vi "Add CSM Module.vi"(6 "Config Path":path, 8 "error in (no error)":errorcluster, 10 "CSM-VI":string, 11 "CSM Name":string) -> (0 "error out":errorcluster)   [LabVIEW 2017, in "CSM-Helper API with lvcsm Support.lvlib"]
uses:
  CSM-Helper API with lvcsm Support.lvlib
  4050c0ca-c03f-4557-9b57-a0dfa28f159e.vi
  <vilib>/Utility/config.llb/Close Config Data.vi
  <vilib>/Utility/config.llb/Write Key.vi
  <vilib>/Utility/config.llb/Write Key (Double).vi
  <vilib>/Utility/config.llb/Write Key (I32).vi
  <vilib>/Utility/config.llb/Write Key (String).vi
  lvcsmFile/Path to lvcsm String.vi
  <vilib>/Utility/config.llb/Remove Key.vi
  <vilib>/Utility/config.llb/Get Key Names.vi
  <vilib>/Utility/Data Type/Get Type Information.vi
  <vilib>/Utility/Data Type/Get Array Information.vi
  <vilib>/Utility/config.llb/Write Key (Boolean).vi
  <vilib>/Utility/config.llb/Open Config Data.vi
  lvcsmFile/lvcsm File Path.vi
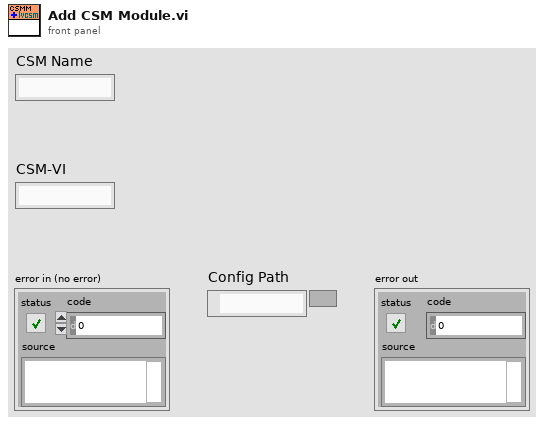
[diagram p1: front panel]
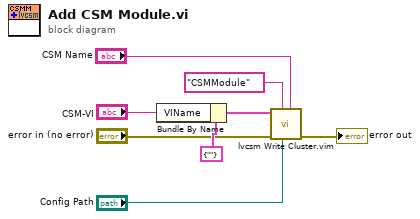
[diagram p0: block diagram]
diagram:
  n1 = Bundle By Name(cluster=cluster{"VIName":string} {"VIName"=""}, "VIName"="CSM-VI") -> (w7:cluster{"VIName":string})
  n2 = call "lvcsm Write Cluster.vim"("Sub-section (\"\")"="CSM Name", "Config Path"="Config Path", "Section"="CSMModule", "Error In"="error in (no error)", "Configuration"=w7) -> ("error out"=→"error out":errorcluster)  [unwired: 6 in]
